vi "Initialize.vi"(7 "Serial Configuration":T1={"Baud Rate"=9600, "Flow Control"=0, "Parity"=0, "Data Bits"=8} {"Flow Control" items=["NONE", "SOFTWARE"]; "Data Bits" items=["7"=7, "8"=8]; "Parity" items=["NONE", "ODD", "EVEN"]; "Baud Rate" items=["300"=300, "600"=600, "1200"=1200, "2400"=2400, "4800"=4800, "9600"=9600, "19200"=19200]}, 8 "error in (no error)":errorcluster, 9 "Reset (True)":bool=TRUE, 10 "ID Query (True)":bool=TRUE, 11 "VISA resource name":refnum<visa-resource-name>) -> (0 "error out":errorcluster, 3 "VISA resource name out":refnum<visa-resource-name>)   [LabVIEW 2025, in "Chroma 19572.lvlib"]
doc: "Establishes communication with the instrument and optionally performs an instrument identification query and/or an instrument reset. It also places the instrument in a default state needed for other instrument driver operations. Therefore, call this VI before calling other instrument driver VIs for this instrument. Generally, you need to call the <b>Initialize</b> VI only once at the beginning of an application."
uses:
  <instrlib>/Chroma 19572/Chroma 19572.lvlib
  <vilib>/ErrorRing/Error Ring.xnode
panel:
  # "(c) 2025 RAMON TABOADA.  ALL RIGHTS RESERVED."
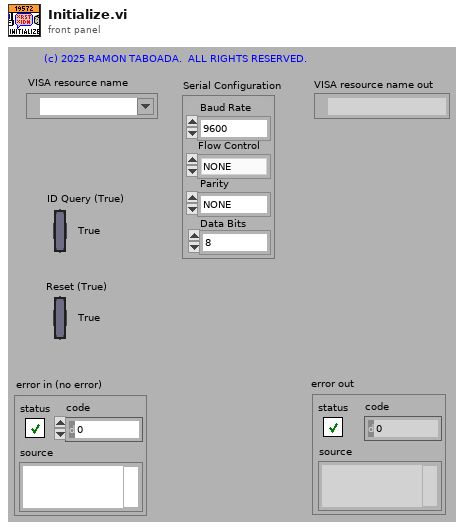
[diagram p1: front panel]
types:
  T1 = cluster{"Baud Rate":u32, "Flow Control":u16, "Parity":u16, "Data Bits":u16}
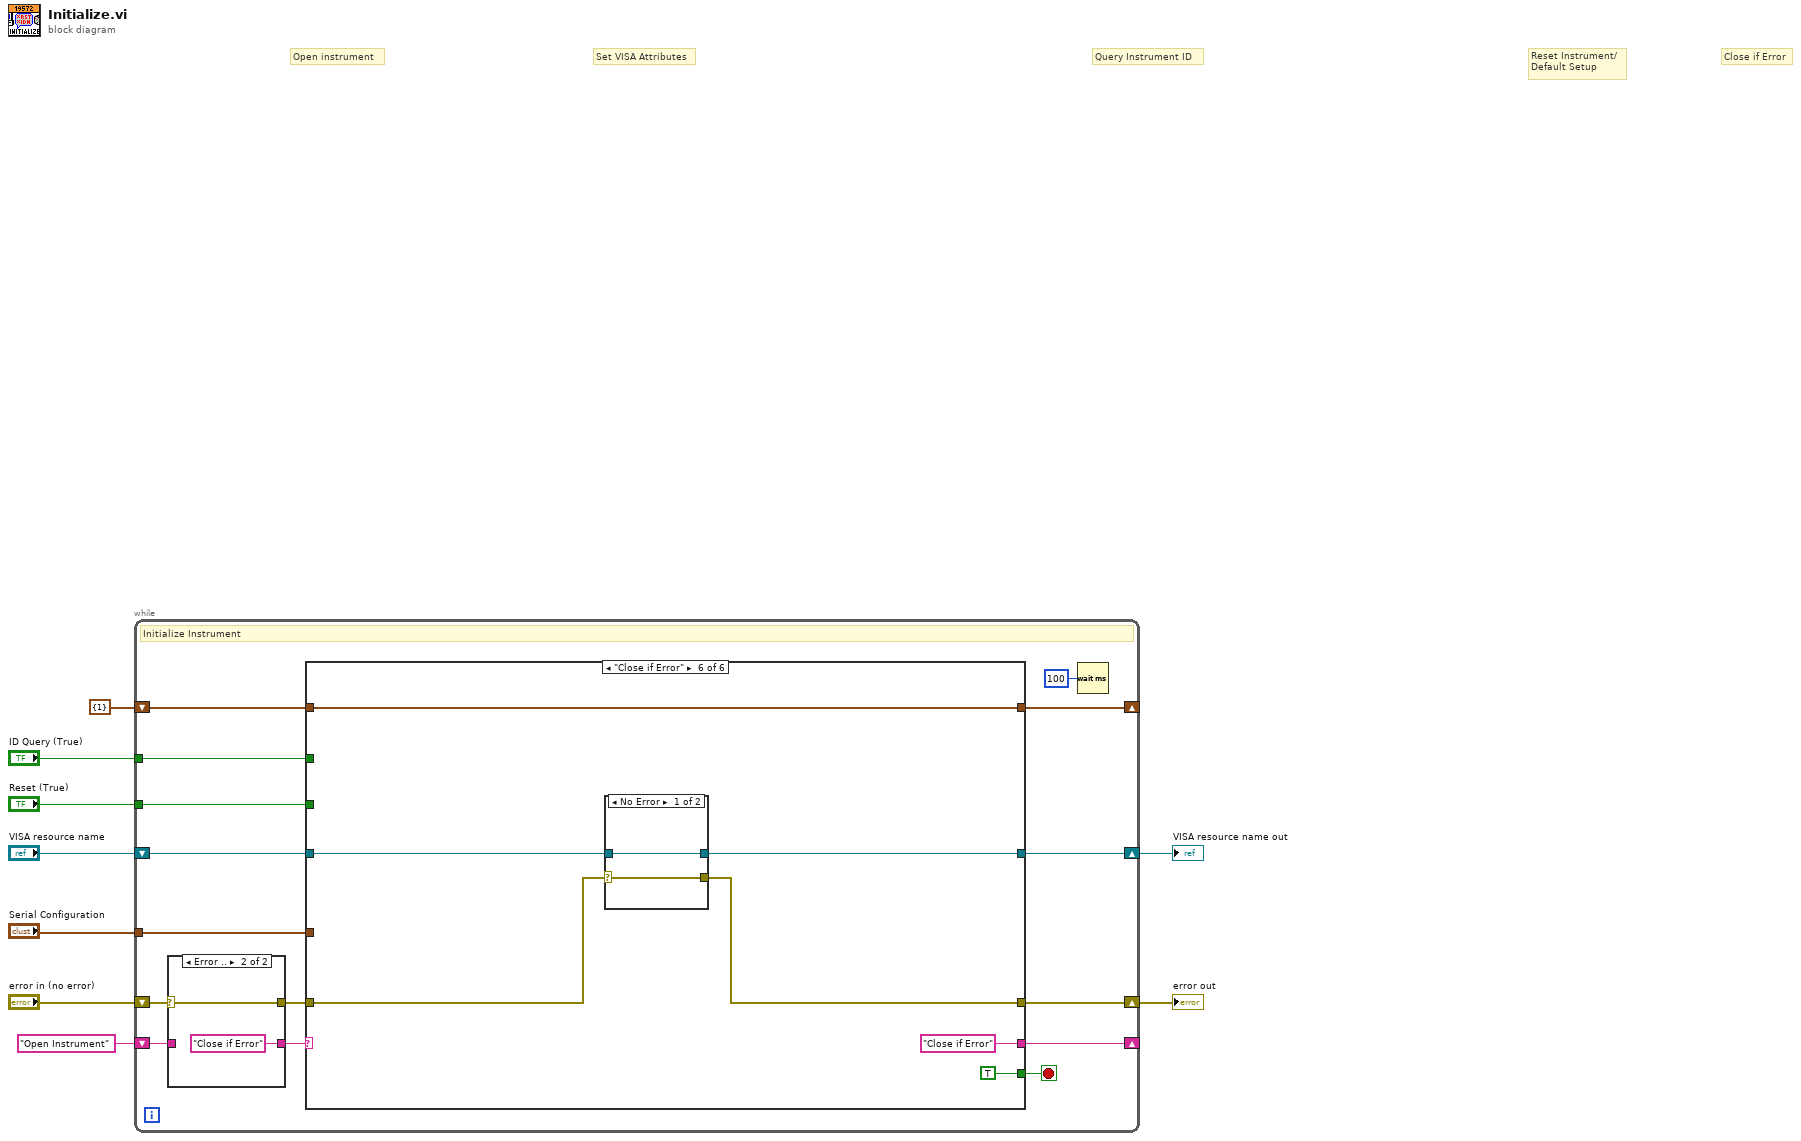
[diagram p0: block diagram]
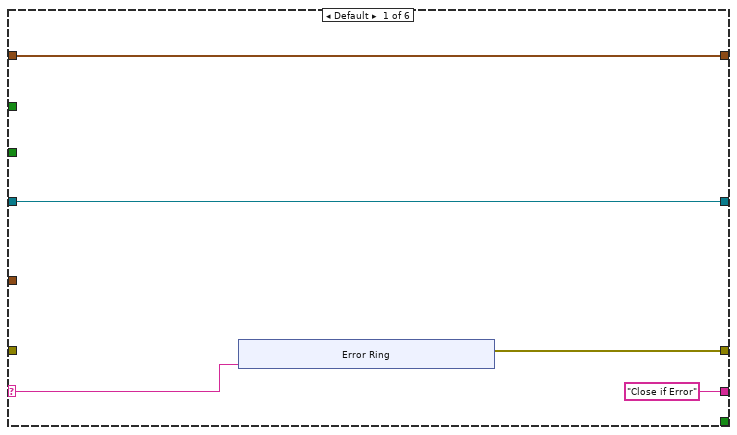
[diagram p3: hidden frame]
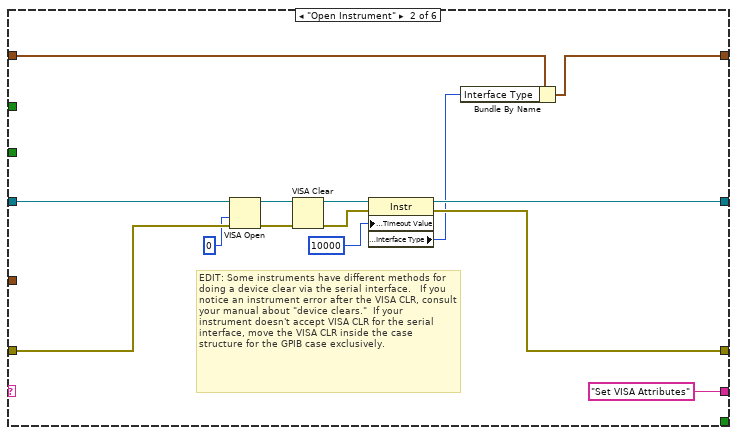
[diagram p4: hidden frame]
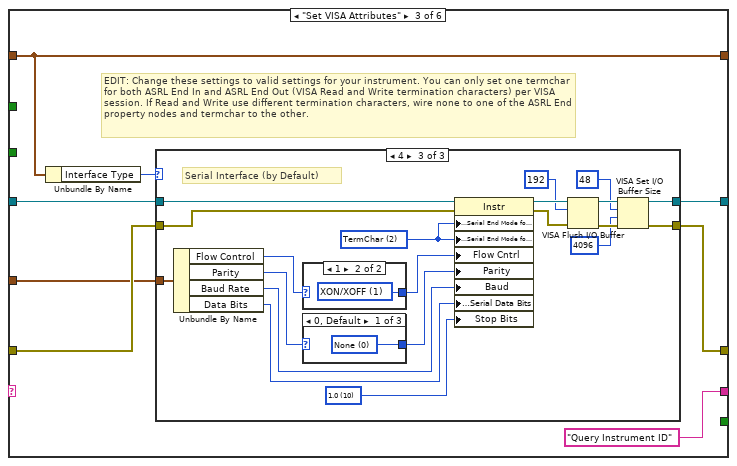
[diagram p5: hidden frame]
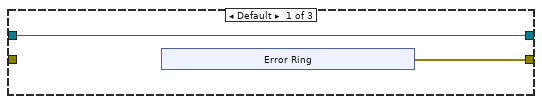
[diagram p6: hidden frame]
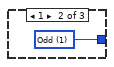
[diagram p8: hidden frame]
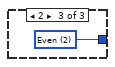
[diagram p9: hidden frame]
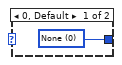
[diagram p10: hidden frame]
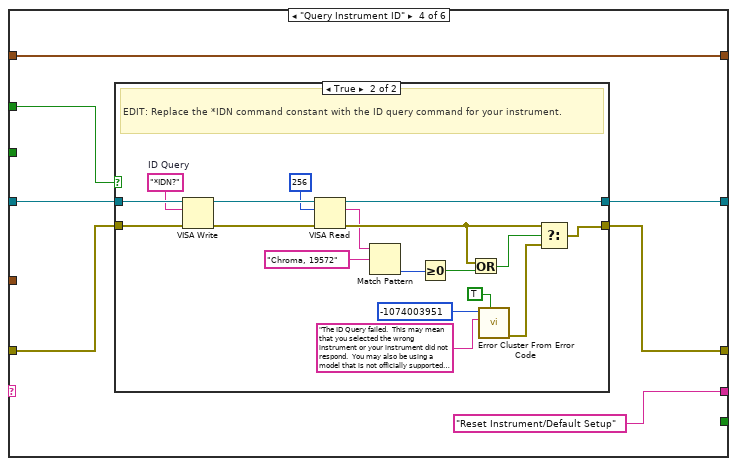
[diagram p11: hidden frame]
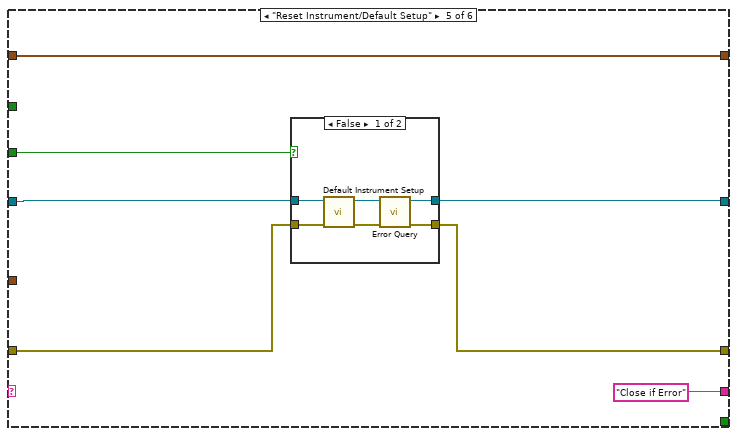
[diagram p13: hidden frame]
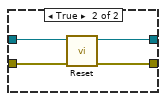
[diagram p14: hidden frame]
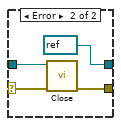
[diagram p15: hidden frame]
diagram:
  # "Set VISA Attributes"
  # "Close if Error"
  # "Query Instrument ID"
  # "Reset Instrument/\nDefault Setup"
  # "Open instrument"
  n1 = while {
    shift-right: [w17] -> w1
    shift-left: "VISA resource name" -> [w18]
    shift-right: [w16] -> w2
    shift-left: "error in (no error)" -> [w23]
    shift-right: [w15] -> _
    shift-left: "Open Instrument" -> [w24]
    tunnel: "ID Query (True)" -> [w19]
    tunnel: "Reset (True)" -> [w20]
    shift-right: [w13] -> _
    shift-left: cluster{"Interface Type":u16} {"Interface Type"=1} -> [w14]
    tunnel: "Serial Configuration" -> [w11]
    stop <- w10 stop-if-true
    # "Initialize Instrument"
    n2 = case shown="Error .." w23 {
      selector: w23 -> [w25 w27]
      tunnel: w24 -> [w26 _]
      tunnel: [w26 "Close if Error"] -> w22
      tunnel: [w25 w27] -> w12
      frame No Error {
      }
      frame Error {
      }
    }
    n3 = case shown="\"Close if Error\"" w22 {
      selector: w22 -> [w32 _ _ _ _ _]
      tunnel: w20 -> [_ _ _ _ w125 _]
      tunnel: w19 -> [_ _ _ w97 _ _]
      tunnel: w18 -> [w33 w49 w62 w102 w129 w146]
      tunnel: [w33 w48 w57 w101 w128 w145] -> w17
      tunnel: [w31 w46 w56 w100 w126 w143] -> w16
      tunnel: ["Close if Error" "Set VISA Attributes" "Query Instrument ID" "Reset Instrument/Default Setup" "Close if Error" "Close if Error"] -> w15
      tunnel: w14 -> [w29 w44 w59 w103 w130 w147]
      tunnel: [w29 w42 w59 w103 w130 w147] -> w13
      tunnel: w12 -> [_ w47 w61 w99 w127 w144]
      tunnel: w11 -> [_ _ w60 _ _ _]
      tunnel: [_ _ _ _ _ TRUE] -> w10
      frame Default {
        n4 = xnode ("Error Ring")("parameter 0"=w32) -> ("error out"=w31:errorcluster)
      }
      frame "Open Instrument" {
        # "EDIT: Some instruments have different methods for doing a device clear via the serial interface.   If you notice an instrument error after the VISA CLR, consult your manual about \"device clears.\"  If your instrument doesn't accept VISA CLR for the serial interface, move the VISA CLR inside the case  structure for the GPIB case exclusively."
        n5 = VISA Open(access mode=u32 0, error in (no error)=w47, VISA resource name=w49) -> (VISA resource name=w53:refnum<visa-resource-name>, error out=w52:errorcluster)  [unwired: 2 in]
        n6 = VISA Clear(VISA resource name=w53, error in (no error)=w52) -> (VISA resource name out=w51:refnum<visa-resource-name>, error out=w50:errorcluster)
        n7 = property class="Instr"(reference=w51, error in=w50, "General Settings:Timeout Value"=u32 10000) -> (reference out=w48:refnum<visa-resource-name>, error out=w46:errorcluster, "Interface Information:Interface Type"=w43:u16)
        n8 = Bundle By Name(cluster=w44, "Interface Type"=w43) -> (w42:cluster{"Interface Type":u16})
      }
      frame "Set VISA Attributes" {
        # "EDIT: Change these settings to valid settings for your instrument. You can only set one termchar for both ASRL End In and ASRL End Out (VISA Read and Write termination characters) per VISA session. If Read and Write use different termination characters, wire none to one of the ASRL End property nodes and termchar to the other."
        n9 = Unbundle By Name(w59) -> ("Interface Type"=w58:u16)
        n10 = case shown="4" w58 {
          tunnel: [w64 w71 w88] -> w57
          tunnel: [w63 w70 w85] -> w56
          tunnel: w62 -> [w64 w71 w90]
          tunnel: w61 -> [_ w70 w91]
          tunnel: w60 -> [_ _ w79]
          frame Default {
            n11 = xnode "Error Ring"() -> ("error out"=w63:errorcluster)
          }
          frame 1 {
            # "GPIB when interface is installed"
          }
          frame 4 {
            w72 = u16 10 items=["1.0"=10, "1.5"=15, "2.0"=20] ("Serial Settings:Stop Bits")
            w80 = u16 2 items=["None", "LastBit", "TermChar"] ("Serial Settings:Serial End Mode for Reads")
            # "Serial Interface (by Default)"
            n12 = Unbundle By Name(w79) -> ("Flow Control"=w78:u16, "Parity"=w76:u16, "Baud Rate"=w74:u32, "Data Bits"=w73:u16)
            n13 = case shown="1" w78 {
              tunnel: [w95 w96] -> w77
              frame 0, Default {
                w95 = u16 0 items=["None", "XON/XOFF", "RTS/CTS", "XON/XOFF & RTS/CTS", "DTR/DSR", "XON/XOFF & DTR/DSR"] ("Serial Settings:Flow Control")
              }
              frame 1 {
                w96 = u16 1 items=["None", "XON/XOFF", "RTS/CTS", "XON/XOFF & RTS/CTS", "DTR/DSR", "XON/XOFF & DTR/DSR"] ("Serial Settings:Flow Control")
              }
            }
            n14 = case shown="0, Default" w76 {
              tunnel: [w92 w93 w94] -> w75
              frame 0, Default {
                w92 = u16 0 items=["None", "Odd", "Even", "Mark", "Space"] ("Serial Settings:Parity")
              }
              frame 1 {
                w93 = u16 1 items=["None", "Odd", "Even", "Mark", "Space"] ("Serial Settings:Parity")
              }
              frame 2 {
                w94 = u16 2 items=["None", "Odd", "Even", "Mark", "Space"] ("Serial Settings:Parity")
              }
            }
            n15 = property class="Instr"(reference=w90, error in=w91, "Serial Settings:Serial End Mode for Reads"=w80, "Serial Settings:Serial End Mode for Writes"=w80, "Flow Cntrl"=w77, "Parity"=w75, "Baud"=w74, "Serial Settings:Serial Data Bits"=w73, "Stop Bits"=w72) -> (reference out=w84:refnum<visa-resource-name>, error out=w87:errorcluster)
            n16 = VISA Flush I/O Buffer(VISA resource name=w84, mask (16)=u16 192, error in (no error)=w87) -> (VISA resource name out=w89:refnum<visa-resource-name>, error out=w86:errorcluster)
            n17 = VISA Set I/O Buffer Size(VISA resource name=w89, mask (16)=u16 48, size (4096)=u32 4096 ("size (0)"), error in (no error)=w86) -> (VISA resource name out=w88:refnum<visa-resource-name>, error out=w85:errorcluster)
          }
        }
      }
      frame "Query Instrument ID" {
        n18 = case shown="True" w97 {
          tunnel: [w104 w123] -> w100
          tunnel: [w105 w120] -> w101
          tunnel: w102 -> [w105 w121]
          tunnel: w99 -> [w104 w122]
          frame False {
          }
          frame True {
            w115 = "*IDN?"  # ID Query
            # "EDIT: Replace the *IDN command constant with the ID query command for your instrument."
            n19 = VISA Write(VISA resource name=w121, write buffer=w115, error in (no error)=w122) -> (VISA resource name out=w119:refnum<visa-resource-name>, error out=w118:errorcluster)  [unwired: 1 out]
            n20 = VISA Read(VISA resource name=w119, byte count=u32 256, error in (no error)=w118) -> (VISA resource name out=w120:refnum<visa-resource-name>, read buffer=w106:string, error out=w108:errorcluster)  [unwired: 1 out]
            n21 = Match Pattern(string=w106, regular expression="Chroma, 19572") -> (offset past match=w110:i32)  [unwired: 1 in, 3 out]
            n22 = Greater Or Equal To 0?(x=w110) -> (x >= 0?=w109:bool)
            n23 = Or(x=w108, y=w109) -> (x .or. y?=w107:bool)
            n24 = call <vilib>:"Error Cluster From Error Code.vi"("show call chain? (False)"=TRUE, "error message (\"\")"="The ID Query failed.  This may mean that you selected the wrong instrument or your instrument did not respond.  You may also be using a model that is not officially supported by this driver.  If you are sure that you have selected the correct instrument and it is responding, try disabling the ID Query." ("Source (VI Name)"), "error code (0)"=-1074003951 ("Code")) -> ("error out"=w114:errorcluster)  [unwired: 6 in]
            n25 = Select(t=w108, s=w107, f=w114) -> (s? t:f=w123:errorcluster)
          }
        }
      }
      frame "Reset Instrument/Default Setup" {
        n26 = case shown="False" w125 {
          tunnel: w127 -> [w135 w137]
          tunnel: [w132 w140] -> w126
          tunnel: w129 -> [w136 w138]
          tunnel: [w133 w139] -> w128
          frame False {
            n27 = call <instrlib>:"Default Instrument Setup.vi"("error in (no error)"=w135, "VISA resource name"=w136) -> ("error out"=w131:errorcluster, "VISA resource name out"=w134:refnum<visa-resource-name>)  [unwired: 8 in]
            n28 = call <instrlib>:"Error Query.vi"("error in (no error)"=w131, "VISA resource name"=w134) -> ("error out"=w132:errorcluster, "VISA resource name out"=w133:refnum<visa-resource-name>)  [unwired: 6 in, 2 out]
          }
          frame True {
            n29 = call <instrlib>:"Reset.vi"("error in (no error)"=w137, "VISA resource name"=w138) -> ("error out"=w140:errorcluster, "VISA resource name out"=w139:refnum<visa-resource-name>)  [unwired: 8 in]
          }
        }
      }
      frame "Close if Error" {
        n30 = case shown="No Error" w144 {
          selector: w144 -> [w148 w151]
          tunnel: w146 -> [w149 w152]
          tunnel: [w149 refnum<visa-resource-name> refnum ("VISA resource name out")] -> w145
          tunnel: [w148 w153] -> w143
          frame No Error {
          }
          frame Error {
            n31 = call <instrlib>:"Close.vi"("error in (no error)"=w151, "VISA resource name"=w152) -> ("error out"=w153:errorcluster)  [unwired: 9 in]
          }
        }
      }
    }
    n32 = Wait (ms)(milliseconds to wait=u32 100) -> ()  [unwired: 1 out]
  }
  "VISA resource name out" <- w1
  "error out" <- w2
